vi "SimpleAdd.vi"() -> ()   [LabVIEW 2020]
panel:
  in  "Number 3":dbl format="%#_13g"
  in  "Number 2":dbl format="%#_13g"
  in  "Number 1":dbl format="%#_13g"
  out "Sum":dbl
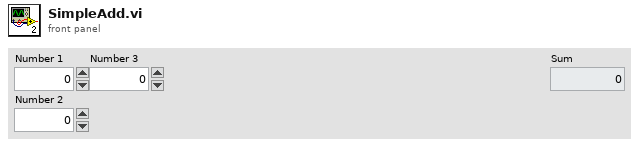
[diagram p1: front panel]
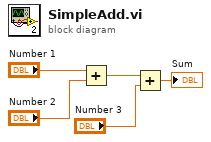
[diagram p0: block diagram]
diagram:
  n1 = Add(x="Number 1", y="Number 2") -> (x+y=w3:dbl)
  n2 = Add(x=w3, y="Number 3") -> (x+y=→"Sum":dbl)
